vi "RefNums_DriverStation.vi"() -> ()   [LabVIEW 2018]
panel:
  out "Joystick 1":string="FrontLeftDrive"
  out "Joystick 0":string="FrontLeftDrive"
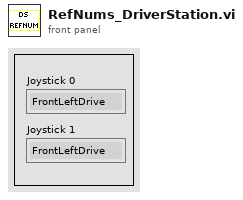
[diagram p1: front panel]
diagram:
